vi "PCO_GetCameraName.vi"(8 "error in (no error)":errorcluster {"code" format="%x"}, 11 "ph":u64) -> (0 "error out":errorcluster {"code" format="%x"}, 1 "szCameraName":string, 2 "ErrorMessage":i32 format="%x", 3 "ph out":u64)   [LabVIEW 2020, in "SDK.lvlib" / "GeneralCameraStatus.lvlib"]
doc: "<b>Description:</b>\nThis function retrieves the name of the camera. A zero terminated ASCII string will be returned in the provided array. This array must be large enough to hold the complete string and the termination value, if not, an error will be returned. At most 40 bytes will be returned from the camera.\n\n<b>Supported camera type:</b>\nAll cameras\n\n<b>Descriptor dependency:</b>\nNone"
uses:
  GeneralCameraStatus.lvlib
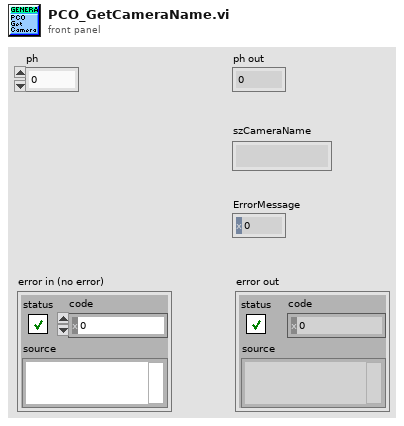
[diagram p1: front panel]
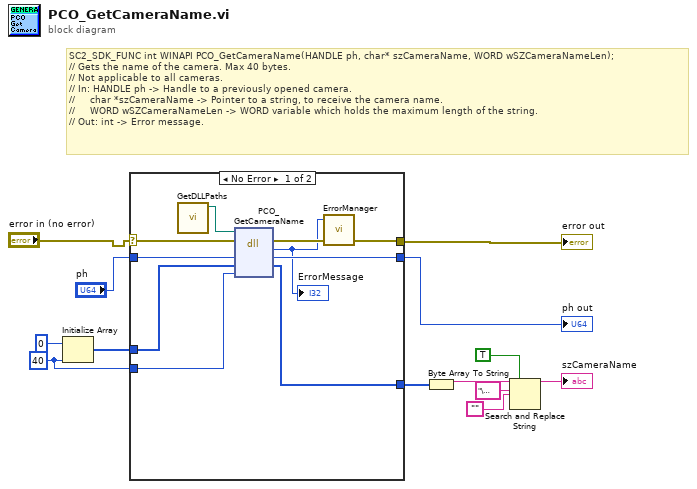
[diagram p0: block diagram]
diagram:
  w8 = u16 40 ("dimension size")
  # "SC2_SDK_FUNC int WINAPI PCO_GetCameraName(HANDLE ph, char* szCameraName, WORD wSZCameraNameLen);\n// Gets the name of the camera. Max 40 bytes.\n// Not applicable to all cameras.\n// In: HANDLE ph -> Handle to a previously opened camera.\n//     char *szCameraName -> Pointer to a string, to receive the camera name.\n//     WORD wSZCameraNameLen -> WORD variable which holds the maximum length of the string.\n// Out: int -> Error message."
  n1 = Initialize Array(u8 0, w8) -> (w7:u8[])
  n2 = case shown="No Error" "error in (no error)" {
    selector: "error in (no error)" -> [w21 w26]
    tunnel: [w22 w26] -> w13
    tunnel: "ph" -> [w20 w25]
    tunnel: [w19 w25] -> w10
    tunnel: w8 -> [w17 _]
    tunnel: w7 -> [w16 w24]
    tunnel: [w15 w24] -> w2
    frame No Error {
      n3 = call "GetDLLPaths.vi"() -> ("SC2_Cam_Path"=w14:path)  [unwired: 9 in, 2 out]
      n4 = dll-call lib="?" fn="PCO_GetCameraName"(path in=w14, error in=w21, "ph"=w20, "szCameraName"=w16, "wSZCameraNameLen"=w17) -> (error out=w23:errorcluster, "return type"=w18:i32, "ph"=w19:u64, "szCameraName"=w15:u8[])  [unwired: 2 in, 1 out]
      "ErrorMessage" <- w18
      n5 = call "ErrorManager.vi"("error in (no error)"=w23, "error code"=w18) -> ("error out"=w22:errorcluster)  [unwired: 3 in]
    }
    frame Error {
    }
  }
  "error out" <- w13
  "ph out" <- w10
  n6 = Byte Array To String(unsigned byte array=w2) -> (string=w6:string)
  n7 = Search and Replace String(replace all?=TRUE ("replace all? (F)"), input string=w6, search string="\u0000", replace string="" ("replace string (\"\")")) -> (result string=→"szCameraName":string)  [unwired: 4 in, 3 out]
